vi "Pre Launch Init.vi"(11 "CS++Nanotec in":refnum<class "CS++Nanotec.lvclass">) -> (0 "error out":errorcluster, 3 "CS++Nanotec out":refnum<class "CS++Nanotec.lvclass">)   [LabVIEW 2015, in "CS++Nanotec.lvlib" / "CS++Nanotec.lvclass"]
doc: "(<B>Filename</B>: Actor Framework.lvlib:Actor.lvclass:Pre Launch Init.vi)\n\nDefines behavior that occurs after the Launch Actor method is invoked but before the actor's Actor Core method begins running.\n\nThe Pre Launch Init method is guaranteed to finish before the Launch Actor method returns to its caller and before the actor itself receives any messages. Any references that the Pre Launch Init method obtains are guaranteed to have the same lifetime as the actor itself. Any errors that the Pre Launch Init method returns will abort the launch.\n\nBy default, this method does nothing. A descendant class may override it to define behavior."
uses:
  CS++Nanotec.lvclass
  CS++Nanotec.lvclass/CS++Nanotec.ctl
  CSPP_DeviceBase/CS++Motor/CS++Motor.lvclass
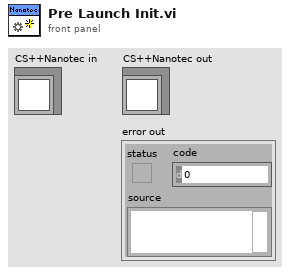
[diagram p1: front panel]
types:
  T1 = cluster{"AxisNumber":u8, "Raw-Position":dbl, "Enum":enum16{"RelativeMovement", "AbsoluteMovement", "Stop", "ReferenceMovement"}}
  T2 = cluster{"Stop":refnum<user-event>, "Pos Update":refnum<user-event>, "Reset":refnum<user-event>}
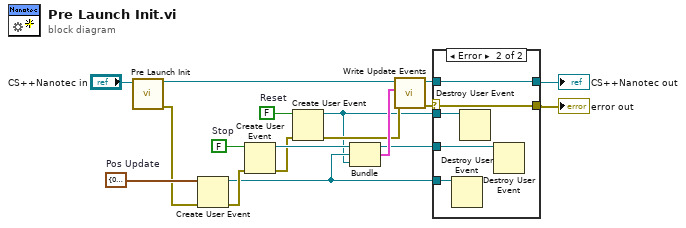
[diagram p0: block diagram]
diagram:
  w8 = FALSE  # Reset
  w9 = T1 {"AxisNumber"=0, "Raw-Position"=0.0, "Enum"=enum."RelativeMovement"}  # Pos Update
  w14 = FALSE  # Stop
  n1 = call-parent "Pre Launch Init.vi"("CS++Motor in"="CS++Nanotec in") -> ("error out"=w1:errorcluster, "CS++Motor out"=w2:refnum<class "CS++Nanotec.lvclass">)  [unwired: 9 in]
  n2 = Create User Event(user event datatype=w9, error in=w1) -> (user event=w10:refnum<user-event>, error out=w11:errorcluster)
  n3 = Create User Event(user event datatype=w14, error in=w11) -> (user event=w12:refnum<user-event>, error out=w7:errorcluster)
  n4 = Create User Event(user event datatype=w8, error in=w7) -> (user event=w5:refnum<user-event>, error out=w6:errorcluster)
  n5 = Bundle("Stop"=w12, "Pos Update"=w10, "Reset"=w5) -> (w13:T2)  [unwired: 1 in]
  n6 = call "Write Update Events.vi"("error in (no error)"=w6, "Update Events"=w13, "CS++Nanotec in"=w2) -> ("error out"=w16:errorcluster, "CS++Nanotec out"=w15:refnum<class "CS++Nanotec.lvclass">)  [unwired: 7 in]
  n7 = case shown="Error" w16 {
    selector: w16 -> [w19 w23]
    tunnel: [w19 w23] -> w3
    tunnel: [w18 w24] -> w4
    tunnel: w15 -> [w18 w24]
    tunnel: w12 -> [_ w22]
    tunnel: w10 -> [_ w21]
    tunnel: w5 -> [_ w20]
    frame No Error {
    }
    frame Error {
      n8 = Destroy User Event(user event=w21) -> ()  [unwired: 1 in, 1 out]
      n9 = Destroy User Event(user event=w20) -> ()  [unwired: 1 in, 1 out]
      n10 = Destroy User Event(user event=w22) -> ()  [unwired: 1 in, 1 out]
    }
  }
  "error out" <- w3
  "CS++Nanotec out" <- w4
